vi "setOperationModeRecursive.vi"(8 "error in (no error)":errorcluster, 10 "Operation Mode in":T1 items=["daqOperationModeTypeUnknown", "daqOperationModeTypeIdle", "daqOperationModeTypeOperation", "daqOperationModeTypeSafeOperation"], 11 "IDevice in":refnum<class "IDevice.lvclass">) -> (0 "error out":errorcluster, 2 "Operation Mode out":T1 items=["daqOperationModeTypeUnknown", "daqOperationModeTypeIdle", "daqOperationModeTypeOperation", "daqOperationModeTypeSafeOperation"], 3 "IDevice out":refnum<class "IDevice.lvclass">)   [LabVIEW 2022 SP3, in "openDAQ.lvlib" / "IBaseObject.lvlib" / "IPropertyObject.lvlib" / "IComponent.lvlib" / "IFolder.lvlib" / "IDevice.lvlib" / "IDevice.lvclass"]
uses:
  <instrlib>/openDAQ/Public/Classes/IDevice/IDevice.lvclass
  <instrlib>/openDAQ/Public/Classes/IDevice/IDevice.lvclass/IDevice.ctl
  <instrlib>/openDAQ/Binaries/Windows/x86/copendaq32.dll
  <instrlib>/openDAQ/Public/TypeDef/daqOperationModeType.ctl
  <instrlib>/openDAQ/openDAQ.lvlib
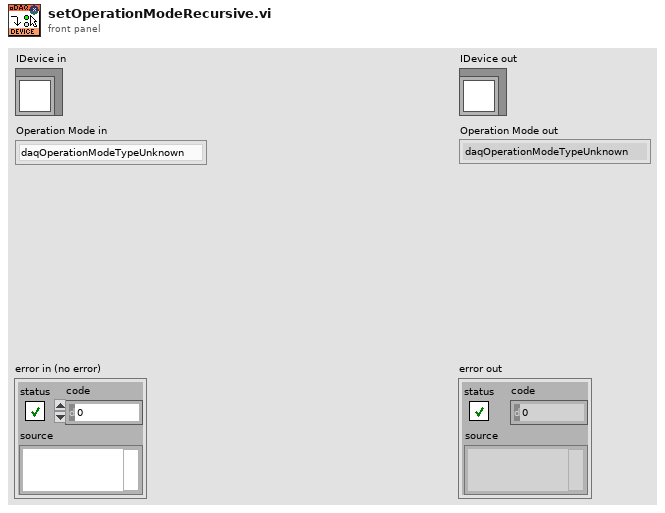
[diagram p1: front panel]
types:
  T1 = typedef "openDAQ.lvlib/daqOperationModeType.ctl" = u16
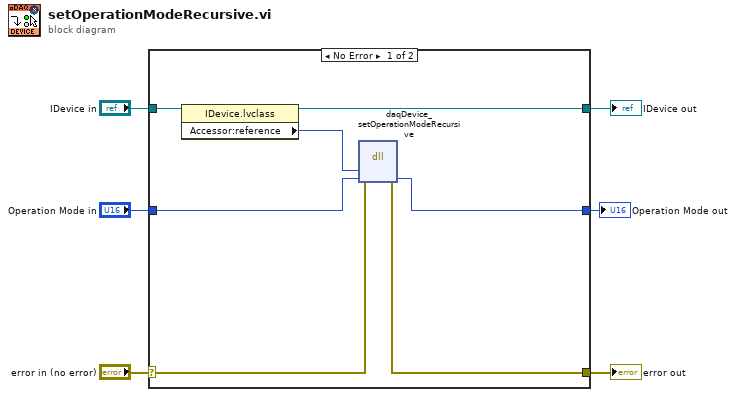
[diagram p0: block diagram]
diagram:
  n1 = case shown="No Error" "error in (no error)" {
    selector: "error in (no error)" -> [w10 w16]
    tunnel: [w9 w16] -> w5
    tunnel: [w11 w15] -> w3
    tunnel: "IDevice in" -> [w13 w15]
    tunnel: "Operation Mode in" -> [w8 w14]
    tunnel: [w7 w14] -> w1
    frame No Error {
      n2 = property class="IDevice.lvclass"(reference=w13) -> (reference out=w11:refnum<class "IDevice.lvclass">, "Accessor:reference"=w12:i64)  [unwired: 1 in, 1 out]
      n3 = dll-call lib="C:/Program Files (x86)/National Instruments/LabVIEW 2022/instr.lib/openDAQ/Binaries/Windows/x86/copendaq*.*" fn="daqDevice_setOperationModeRecursive"(error in=w10, "device"=w12, "operationMode"=w8) -> (error out=w9:errorcluster, "operationMode"=w7:i64)  [unwired: 4 in, 1 out]
    }
    frame Error {
    }
  }
  "error out" <- w5
  "IDevice out" <- w3
  "Operation Mode out" <- w1
